vi "LineWidthFilter3.vi"(0 "X max":i32=22, 1 "X min":i32=4, 2 "Y Max":i32=22, 3 "Y Min":i32=4, 5 "Image Pixels (U8) 2":u8[][](array[numeric])) -> (4 "Image Pixels (U8)":u8[][](array[numeric]))   [LabVIEW 2009]
panel:
  out "Waveform Graph 4":u8[](graph)
  out "Waveform Graph 3":u8[](graph)
  out "Waveform Graph":u8[](graph)
  out "Waveform Graph 2":u8[](graph)
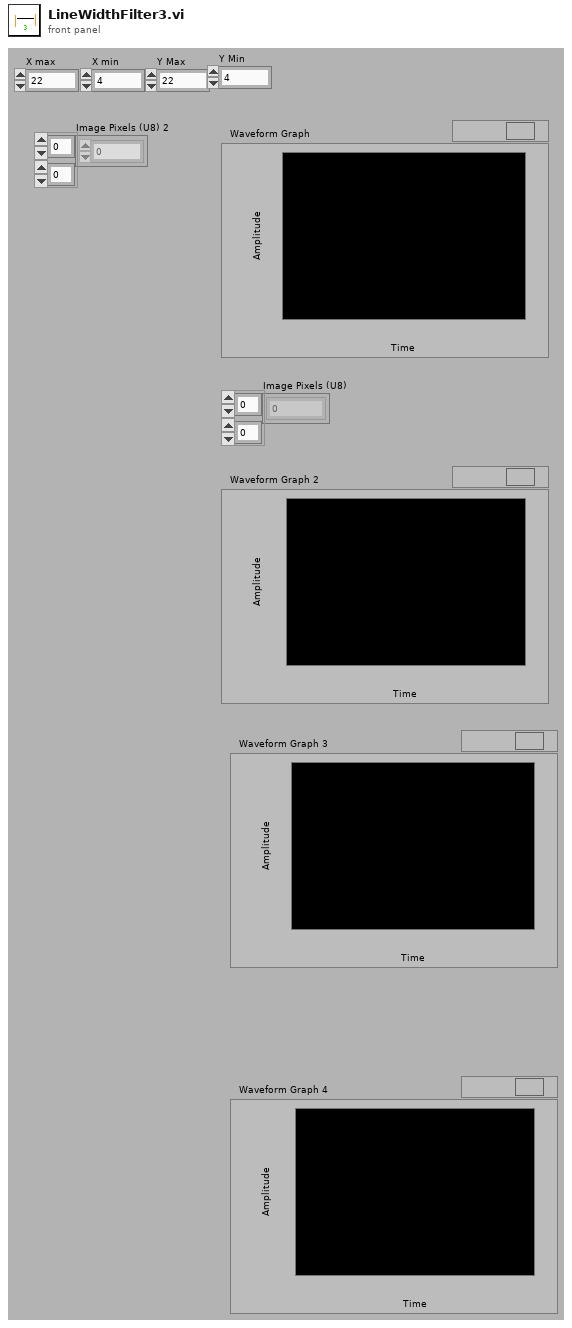
[diagram p1: front panel]
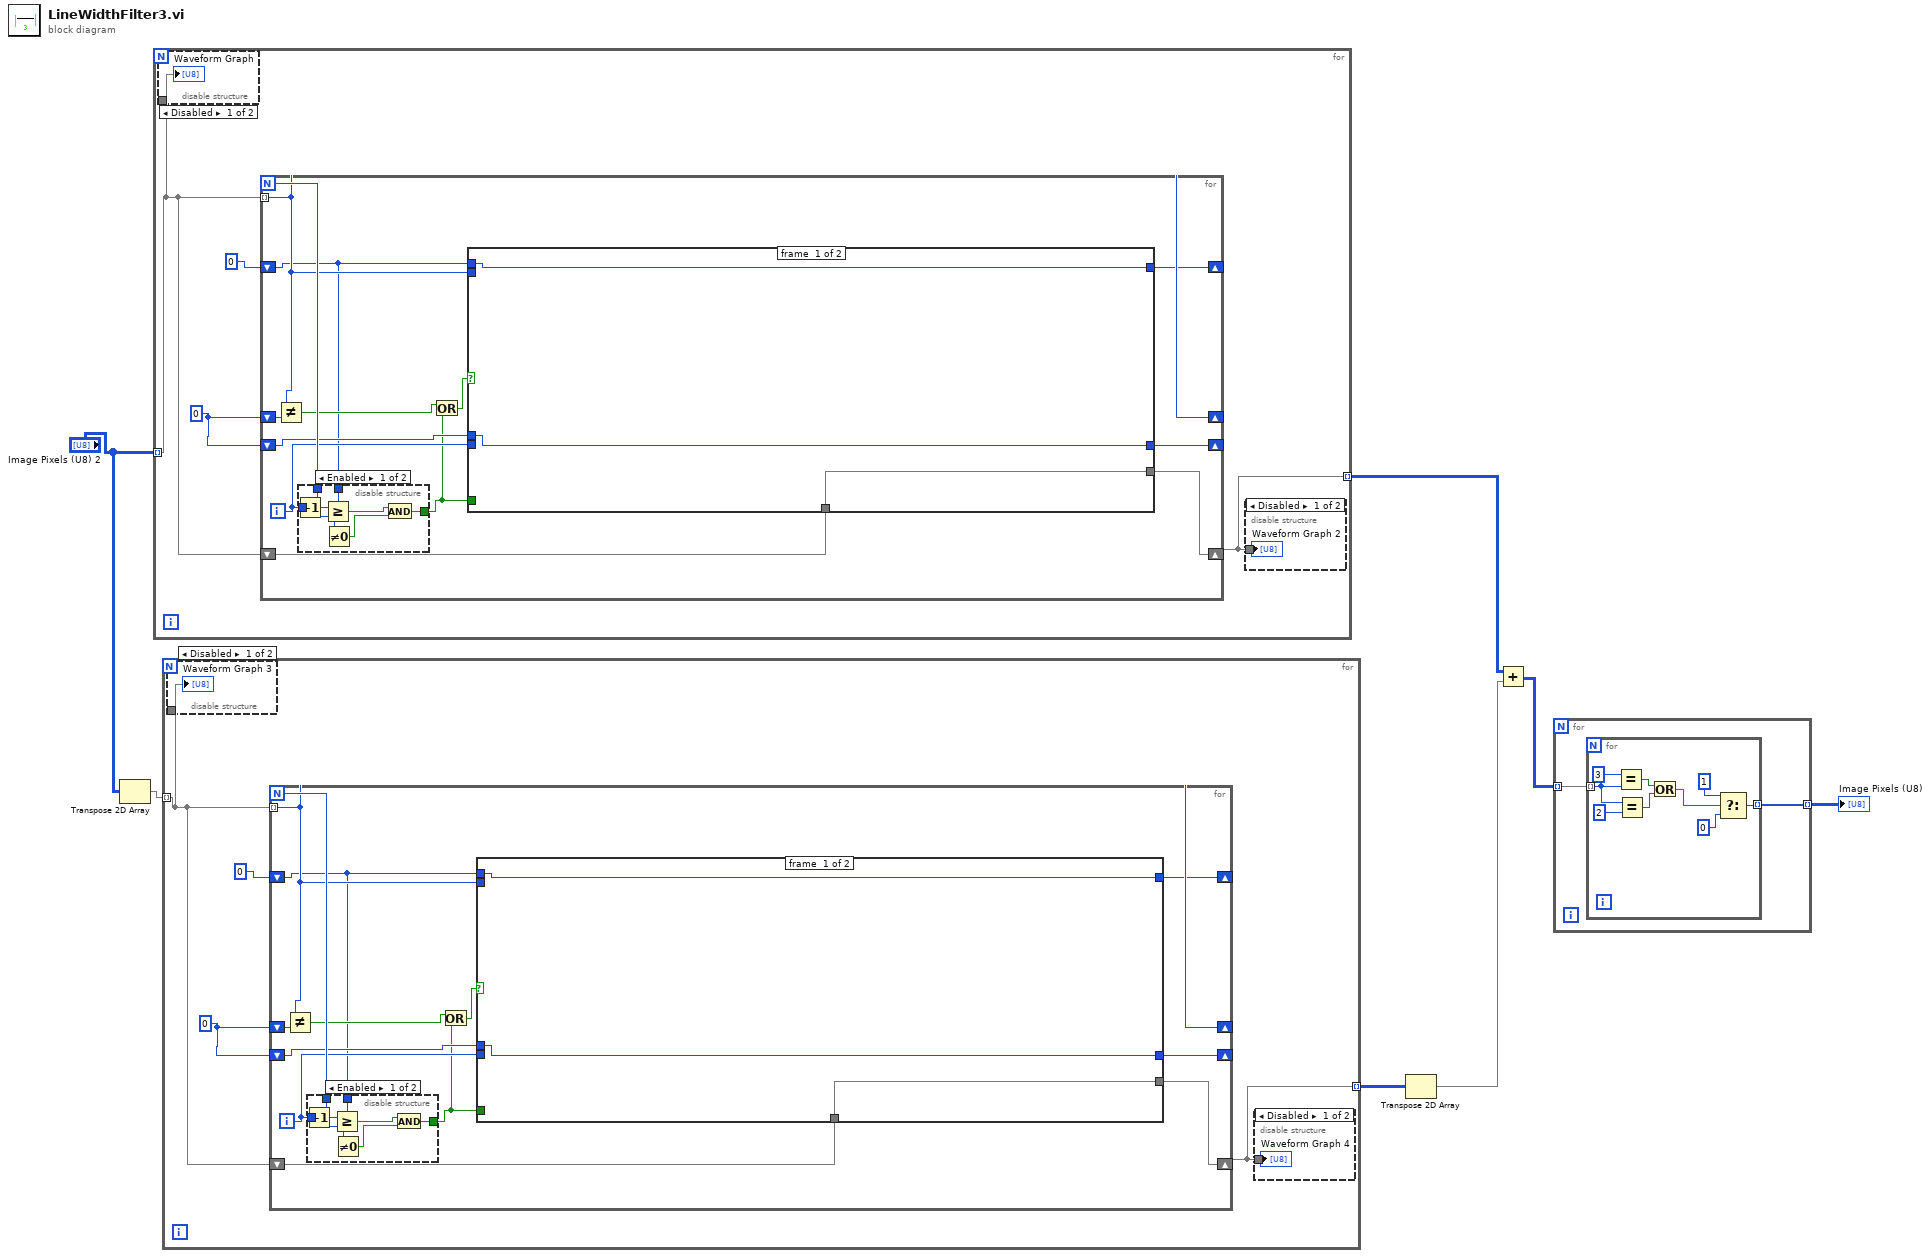
[diagram p0: block diagram]
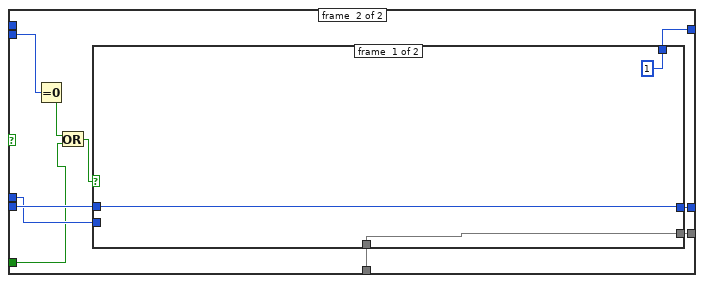
[diagram p4: hidden frame]
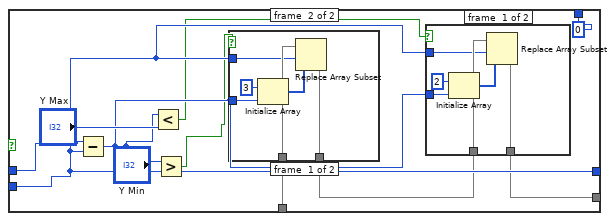
[diagram p5: hidden frame]
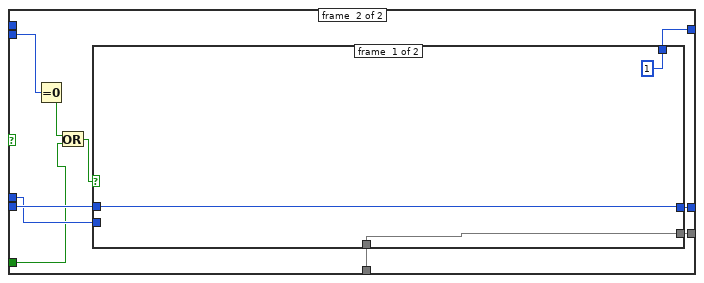
[diagram p11: hidden frame]
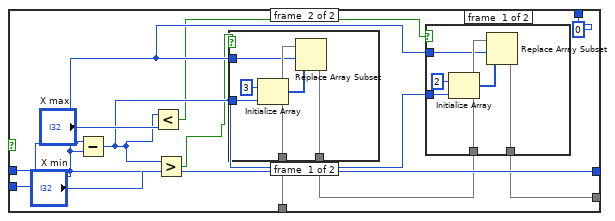
[diagram p12: hidden frame]
diagram:
  n1 = Transpose 2D Array(2D array="Image Pixels (U8) 2") -> (transposed array=w4:u8[][])
  n2 = for {
    tunnel: "Image Pixels (U8) 2" -> [w10] mode=indexing
    tunnel: [w9] -> w5 mode=indexing
    w11 = u8 0
    n3 = disable-structure shown="Disabled" {
      disable-tunnel: w10 -> [w12 _]
      frame #0 {
        "Waveform Graph" <- w12
      }
      frame #1 {
      }
    }
    n4 = for {
      N -> [w22]
      tunnel: w10 -> [w19] mode=indexing
      shift-right: [w19] -> _
      shift-left: w11 -> [w26]
      shift-right: [w25] -> _
      shift-left: w11 -> [w20]
      shift-right: [w23] -> w9
      shift-left: w10 -> [w24]
      shift-right: [w15] -> _
      shift-left: u8 0 -> [w14]
      i -> [w21]
      n5 = Not Equal?(x=w19, y=w26) -> (x != y?=w18:bool)
      n6 = disable-structure shown="Enabled" {
        disable-tunnel: w21 -> [w74 _]
        disable-tunnel: w22 -> [w70 _]
        disable-tunnel: [w69 _] -> w17
        disable-tunnel: w14 -> [w68 _]
        frame #0 {
          n7 = Increment(x=w74) -> (x+1=w73:i32)
          n8 = Greater Or Equal?(x=w73, y=w70) -> (x >= y?=w72:bool)
          n9 = Not Equal To 0?(x=w68) -> (x != 0?=w71:bool)
          n10 = And(x=w72, y=w71) -> (x .and. y?=w69:bool)
        }
        frame #1 {
        }
      }
      n11 = Or(x=w18, y=w17) -> (x .or. y?=w16:bool)
      n12 = case shown="True" w16 {
        tunnel: [w28 w39] -> w25
        tunnel: w24 -> [w29 w38]
        tunnel: [w29 w37] -> w23
        tunnel: w21 -> [_ w36]
        tunnel: w20 -> [w28 w35]
        tunnel: w19 -> [_ w34]
        tunnel: w17 -> [_ w32]
        tunnel: w14 -> [w27 _]
        tunnel: [w27 w30] -> w15
        frame #0 {
        }
        frame #1 {
          n13 = Equal To 0?(x=w34) -> (x = 0?=w33:bool)
          n14 = Or(x=w33, y=w32) -> (x .or. y?=w31:bool)
          n15 = case shown="True" w31 {
            tunnel: [w41 w49] -> w39
            tunnel: w36 -> [w41 w53]
            tunnel: w35 -> [_ w49]
            tunnel: w38 -> [w42 w52]
            tunnel: [w42 w46] -> w37
            tunnel: [u8 1 u8 0] -> w30
            frame #0 {
            }
            frame #1 {
              n16 = Subtract(x=w53, y=w49) -> (x-y=w48:i32)
              n17 = Less?(x=w48, y="X max") -> (x < y?=w44:bool)
              n18 = Greater?(x=w48, y="X min") -> (0:w45:bool)
              n19 = case shown="False" w45 {
                tunnel: w52 -> [w66 w67]
                tunnel: w48 -> [w65 _]
                tunnel: w49 -> [w62 _]
                tunnel: [w61 w67] -> w47
                frame #0 {
                  n20 = Initialize Array(u8 3 ("element"), w65) -> (w63:u8[])
                  n21 = Replace Array Subset(array=w66, new element=w63, index=w62) -> (w61:u8[])
                }
                frame #1 {
                }
              }
              n22 = case shown="False" w44 {
                tunnel: w47 -> [w59 w60]
                tunnel: w48 -> [w58 _]
                tunnel: w49 -> [w55 _]
                tunnel: [w54 w60] -> w46
                frame #0 {
                  n23 = Initialize Array(u8 2 ("element"), w58) -> (w56:u8[])
                  n24 = Replace Array Subset(array=w59, new element=w56, index=w55) -> (w54:u8[])
                }
                frame #1 {
                }
              }
            }
          }
        }
      }
    }
    n25 = disable-structure shown="Disabled" {
      disable-tunnel: w9 -> [w13 _]
      frame #0 {
        "Waveform Graph 2" <- w13
      }
      frame #1 {
      }
    }
  }
  n26 = for {
    tunnel: w4 -> [w77] mode=indexing
    tunnel: [w76] -> w3 mode=indexing
    w78 = u8 0
    n27 = disable-structure shown="Disabled" {
      disable-tunnel: w77 -> [w79 _]
      frame #0 {
        "Waveform Graph 3" <- w79
      }
      frame #1 {
      }
    }
    n28 = for {
      N -> [w89]
      tunnel: w77 -> [w86] mode=indexing
      shift-right: [w86] -> _
      shift-left: w78 -> [w93]
      shift-right: [w92] -> _
      shift-left: w78 -> [w87]
      shift-right: [w90] -> w76
      shift-left: w77 -> [w91]
      shift-right: [w82] -> _
      shift-left: u8 0 -> [w81]
      i -> [w88]
      n29 = Not Equal?(x=w86, y=w93) -> (x != y?=w85:bool)
      n30 = disable-structure shown="Enabled" {
        disable-tunnel: w88 -> [w141 _]
        disable-tunnel: w89 -> [w137 _]
        disable-tunnel: [w136 _] -> w84
        disable-tunnel: w81 -> [w135 _]
        frame #0 {
          n31 = Increment(x=w141) -> (x+1=w140:i32)
          n32 = Greater Or Equal?(x=w140, y=w137) -> (x >= y?=w139:bool)
          n33 = Not Equal To 0?(x=w135) -> (x != 0?=w138:bool)
          n34 = And(x=w139, y=w138) -> (x .and. y?=w136:bool)
        }
        frame #1 {
        }
      }
      n35 = Or(x=w85, y=w84) -> (x .or. y?=w83:bool)
      n36 = case shown="True" w83 {
        tunnel: [w95 w106] -> w92
        tunnel: w91 -> [w96 w105]
        tunnel: [w96 w104] -> w90
        tunnel: w88 -> [_ w103]
        tunnel: w87 -> [w95 w102]
        tunnel: w86 -> [_ w101]
        tunnel: w84 -> [_ w99]
        tunnel: w81 -> [w94 _]
        tunnel: [w94 w97] -> w82
        frame #0 {
        }
        frame #1 {
          n37 = Equal To 0?(x=w101) -> (x = 0?=w100:bool)
          n38 = Or(x=w100, y=w99) -> (x .or. y?=w98:bool)
          n39 = case shown="True" w98 {
            tunnel: [w108 w116] -> w106
            tunnel: w103 -> [w108 w120]
            tunnel: w102 -> [_ w116]
            tunnel: w105 -> [w109 w119]
            tunnel: [w109 w113] -> w104
            tunnel: [u8 1 u8 0] -> w97
            frame #0 {
            }
            frame #1 {
              n40 = Subtract(x=w120, y=w116) -> (x-y=w115:i32)
              n41 = Less?(x=w115, y="Y Max") -> (x < y?=w111:bool)
              n42 = Greater?(x=w115, y="Y Min") -> (0:w112:bool)
              n43 = case shown="False" w112 {
                tunnel: w119 -> [w133 w134]
                tunnel: w115 -> [w132 _]
                tunnel: w116 -> [w129 _]
                tunnel: [w128 w134] -> w114
                frame #0 {
                  n44 = Initialize Array(u8 3 ("element"), w132) -> (w130:u8[])
                  n45 = Replace Array Subset(array=w133, new element=w130, index=w129) -> (w128:u8[])
                }
                frame #1 {
                }
              }
              n46 = case shown="False" w111 {
                tunnel: w114 -> [w126 w127]
                tunnel: w115 -> [w125 _]
                tunnel: w116 -> [w122 _]
                tunnel: [w121 w127] -> w113
                frame #0 {
                  n47 = Initialize Array(u8 2 ("element"), w125) -> (w123:u8[])
                  n48 = Replace Array Subset(array=w126, new element=w123, index=w122) -> (w121:u8[])
                }
                frame #1 {
                }
              }
            }
          }
        }
      }
    }
    n49 = disable-structure shown="Disabled" {
      disable-tunnel: w76 -> [w80 _]
      frame #0 {
        "Waveform Graph 4" <- w80
      }
      frame #1 {
      }
    }
  }
  n50 = Transpose 2D Array(2D array=w3) -> (transposed array=w6:u8[][])
  n51 = Add(x=w5, y=w6) -> (x+y=w2:u8[][])
  n52 = for {
    tunnel: w2 -> [w143] mode=indexing
    tunnel: [w142] -> w1 mode=indexing
    n53 = for {
      tunnel: w143 -> [w149] mode=indexing
      tunnel: [w150] -> w142 mode=indexing
      n54 = Equal?(x=u8 3, y=w149) -> (x = y?=w146:bool)
      n55 = Equal?(x=w149, y=u8 2) -> (x = y?=w145:bool)
      n56 = Or(x=w146, y=w145) -> (x .or. y?=w144:bool)
      n57 = Select(t=u8 1, s=w144, f=u8 0) -> (s? t:f=w150:u8)
    }
  }
  "Image Pixels (U8)" <- w1
